vi "Test unzip.vi"() -> (0 "error out":errorcluster)   [LabVIEW 2011]
uses:
  <vilib>/zip/NI_Unzip.lvlib
panel:
  in  "Zip file":path
  in  "Target directory (same as Zip file if empty)":path
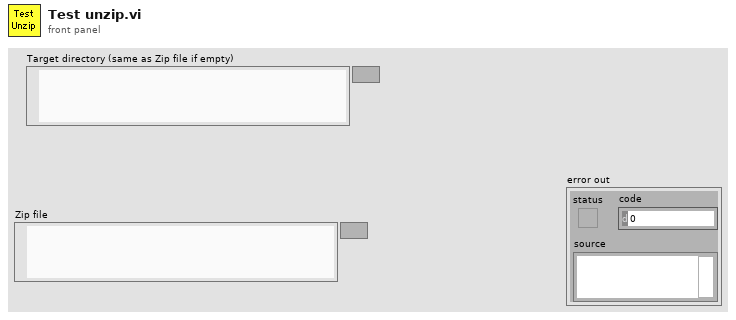
[diagram p1: front panel]
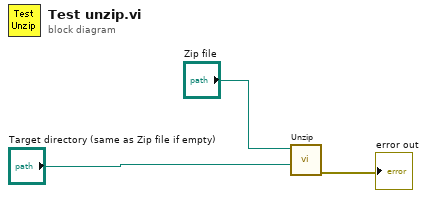
[diagram p0: block diagram]
diagram:
  n1 = call <vilib>:"Unzip.vi"("Target directory (same as Zip file if empty)"="Target directory (same as Zip file if empty)", "Zip file"="Zip file") -> ("error out"=→"error out":errorcluster)  [unwired: 7 in, 2 out]
